vi "Initialize iHR320.vi"(6 "Force Init (F)":bool, 8 "error in (no error)":errorcluster, 9 "Mono ID":string, 10 "Unique ID":string="Mono1", 11 "Spectrometer iHR320 In":refnum<class "Spectrometer iHR320.lvclass">) -> (0 "error out":errorcluster, 2 "Refnum out":refnum<k7> caption="Mono RefNum out", 3 "Spectrometer iHR320 Out":refnum<class "Spectrometer iHR320.lvclass">)   [LabVIEW 2009, in "Spectrometer iHR320.lvclass"]
doc: "Initializes a JY Monochromator/Spectrometer based off of its Unique ID (Mono1,Mono2,...) and returns the Reference Number to the associated ActiveX object.\n\nMono ID is an arbitrary name for the spectrometer."
uses:
  Spectrometer iHR320.lvclass
  Spectrometer iHR320.lvclass/Spectrometer iHR320.ctl
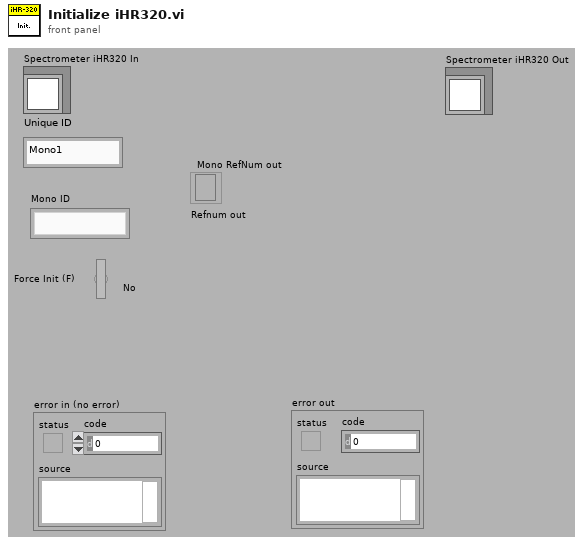
[diagram p1: front panel]
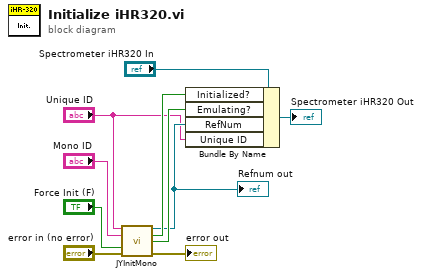
[diagram p0: block diagram]
diagram:
  n1 = call "JYInitMono.vi"("Unique ID"="Unique ID", "Mono ID"="Mono ID", "Force Init"="Force Init (F)", "error in (no error)"="error in (no error)") -> ("Mono RefNum out"=w2:refnum<k7>, "Initialized"=w4:bool, "Emulating"=w3:bool, "error out"=→"error out":errorcluster)  [unwired: 7 in, 1 out]
  "Refnum out" <- w2
  n2 = Bundle By Name(cluster="Spectrometer iHR320 In", "Initialized?"=w4, "Emulating?"=w3, "RefNum"=w2, "Unique ID"="Unique ID") -> (→"Spectrometer iHR320 Out":refnum<class "Spectrometer iHR320.lvclass">)
